vi "X.vi"(9 "X(k-1)":dbl=0.1, 10 "Ýterasyon Denge":dbl, 11 "denge degeri":dbl) -> (0 "error":bool, 2 "output X(k-1)":dbl=0.1, 3 "output x 1":dbl, 4 "cycle":bool)   [LabVIEW 2014]
uses:
  Sub_VI/show_sensitivity.vi
  Sub_VI/global get findinput.vi
  DB_Global_4_kart-Test.vi
panel:
  out "cycle 2":bool
  in  "GPIB In":refnum<visa-resource-name>="GPIB0::8::INSTR"
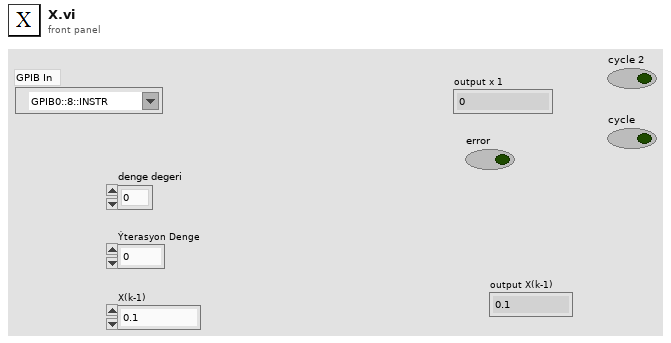
[diagram p1: front panel]
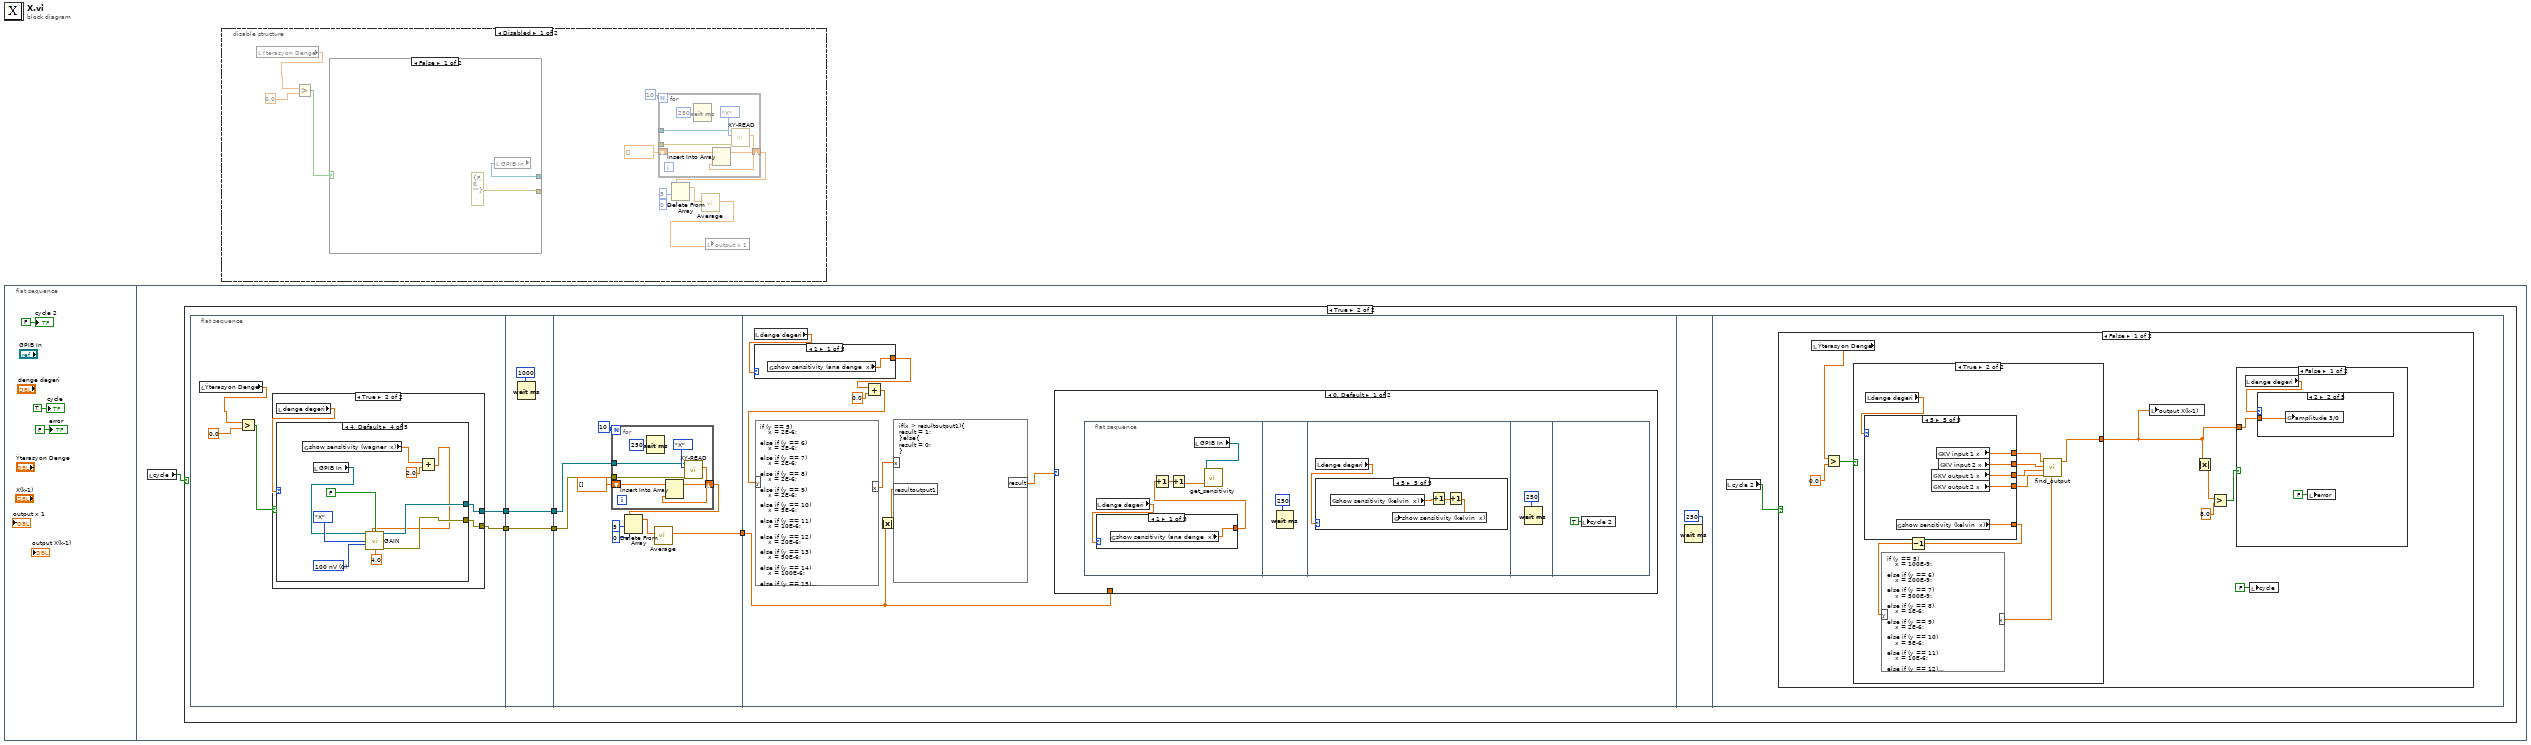
[diagram p0: block diagram]
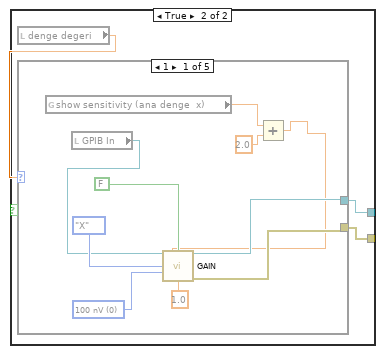
[diagram p2: hidden frame]
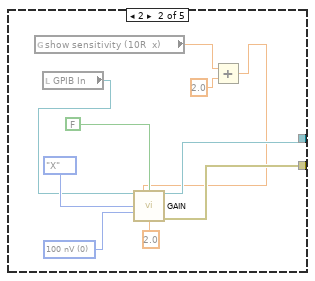
[diagram p3: hidden frame]
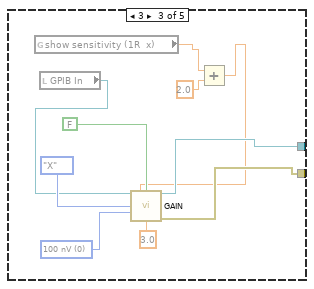
[diagram p4: hidden frame]
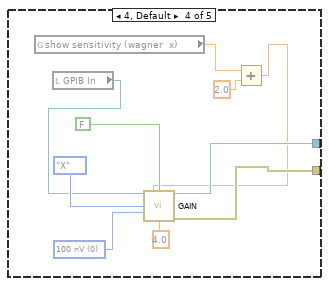
[diagram p5: hidden frame]
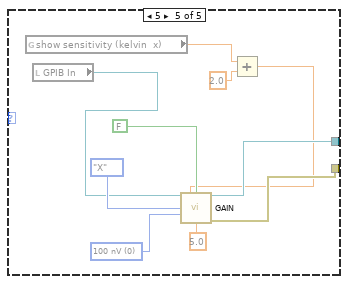
[diagram p6: hidden frame]
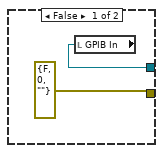
[diagram p9: hidden frame]
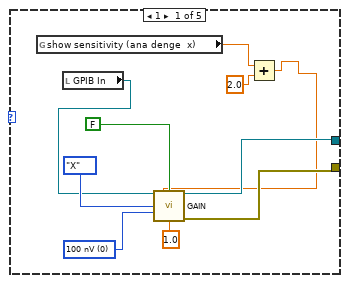
[diagram p10: hidden frame]
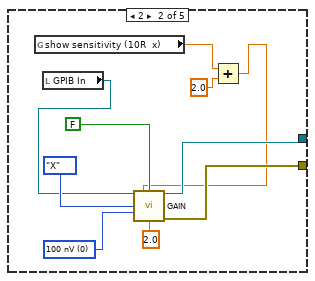
[diagram p11: hidden frame]
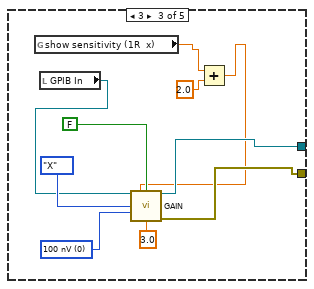
[diagram p12: hidden frame]
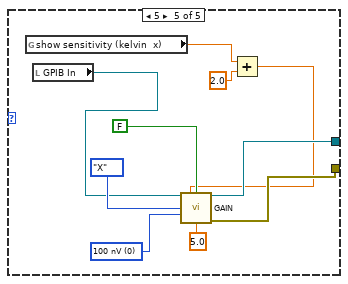
[diagram p13: hidden frame]
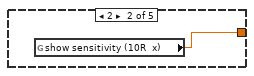
[diagram p14: hidden frame]
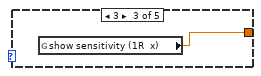
[diagram p15: hidden frame]
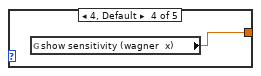
[diagram p16: hidden frame]
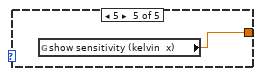
[diagram p17: hidden frame]
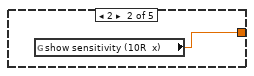
[diagram p18: hidden frame]
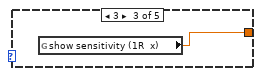
[diagram p19: hidden frame]
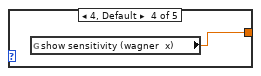
[diagram p20: hidden frame]
diagram:
  n1 = flat-sequence {
    frame #0 {
      "error" <- FALSE ("error")
      "cycle" <- TRUE ("error")
      "cycle 2" <- FALSE ("error")
    }
    frame #1 {
      n2 = local read "cycle"() -> (w4:bool)
      n3 = case shown="True" w4 {
        frame False {
        }
        frame True {
          n4 = flat-sequence {
            tunnel: [w11] -> w8
            tunnel: [w10] -> w6
            tunnel: [w71] -> w9
            tunnel: w8 -> [w71]
            tunnel: [w70] -> w7
            tunnel: w6 -> [w70]
            tunnel: w9 -> [w75]
            tunnel: w7 -> [w74]
            tunnel: [w73] -> w5
            tunnel: w5 -> [w92]
            frame #0 {
              n5 = local read "Ýterasyon Denge"() -> (w12:dbl)
              n6 = Greater?(x=w12, y=0.0) -> (0:w13:bool)
              n7 = case shown="True" w13 {
                tunnel: [w16 w18] -> w11
                tunnel: [errorcluster {"status"=FALSE, "code"=0, "source"=""} ("error out") w17] -> w10
                frame False {
                  n8 = local read "GPIB In"() -> (w16:refnum<visa-resource-name>)
                }
                frame True {
                  n9 = local read "denge degeri"() -> (w19:dbl)
                  n10 = case shown="4, Default" w19 {
                    tunnel: [w24 w34 w44 w54 w65] -> w18
                    tunnel: [w23 w33 w43 w53 w64] -> w17
                    frame 1 {
                      w26 = u16 0 items=["100 nV", "200 nV", "500 nV", "1 uV", "2 uV", "5 uV", "10 uV", "20 uV", "50 uV", "100 uV", "200 uV", "500 uV", "1 mV"] ("Min. Hassasiyet")
                      n11 = global read "show_sensitivity.vi" "show sensitivity (ana denge  x)"() -> (w21:dbl)
                      n12 = local read "GPIB In"() -> (w27:refnum<visa-resource-name>)
                      n13 = Add(x=w21, y=2.0) -> (x+y=w20:dbl)
                      n14 = call "GAIN.vi"("SR850 GPIB In"=w27, "Max. Hassasiyet"=w20, "Auto Gain (False)"=FALSE, "Enum"=enum16{"X", "Y"}."X", "Min. Hassasiyet"=w26, "choose"=1.0) -> ("SR850 GPIB Out"=w24:refnum<visa-resource-name>, "error out"=w23:errorcluster)  [unwired: 7 in, 1 out]
                    }
                    frame 2 {
                      w36 = u16 0 items=["100 nV", "200 nV", "500 nV", "1 uV", "2 uV", "5 uV", "10 uV", "20 uV", "50 uV", "100 uV", "200 uV", "500 uV", "1 mV"] ("Min. Hassasiyet")
                      n15 = global read "show_sensitivity.vi" "show sensitivity (10R  x)"() -> (w30:dbl)
                      n16 = local read "GPIB In"() -> (w37:refnum<visa-resource-name>)
                      n17 = Add(x=w30, y=2.0) -> (x+y=w31:dbl)
                      n18 = call "GAIN.vi"("SR850 GPIB In"=w37, "Max. Hassasiyet"=w31, "Auto Gain (False)"=FALSE, "Enum"=enum16{"X", "Y"}."X", "Min. Hassasiyet"=w36, "choose"=2.0) -> ("SR850 GPIB Out"=w34:refnum<visa-resource-name>, "error out"=w33:errorcluster)  [unwired: 7 in, 1 out]
                    }
                    frame 3 {
                      w46 = u16 0 items=["100 nV", "200 nV", "500 nV", "1 uV", "2 uV", "5 uV", "10 uV", "20 uV", "50 uV", "100 uV", "200 uV", "500 uV", "1 mV"] ("Min. Hassasiyet")
                      n19 = global read "show_sensitivity.vi" "show sensitivity (1R  x)"() -> (w41:dbl)
                      n20 = local read "GPIB In"() -> (w47:refnum<visa-resource-name>)
                      n21 = Add(x=w41, y=2.0) -> (x+y=w40:dbl)
                      n22 = call "GAIN.vi"("SR850 GPIB In"=w47, "Max. Hassasiyet"=w40, "Auto Gain (False)"=FALSE, "Enum"=enum16{"X", "Y"}."X", "Min. Hassasiyet"=w46, "choose"=3.0) -> ("SR850 GPIB Out"=w44:refnum<visa-resource-name>, "error out"=w43:errorcluster)  [unwired: 7 in, 1 out]
                    }
                    frame 4, Default {
                      w56 = u16 0 items=["100 nV", "200 nV", "500 nV", "1 uV", "2 uV", "5 uV", "10 uV", "20 uV", "50 uV", "100 uV", "200 uV", "500 uV", "1 mV"] ("Min. Hassasiyet")
                      n23 = global read "show_sensitivity.vi" "show sensitivity (wagner  x)"() -> (w51:dbl)
                      n24 = local read "GPIB In"() -> (w57:refnum<visa-resource-name>)
                      n25 = Add(x=w51, y=2.0) -> (x+y=w50:dbl)
                      n26 = call "GAIN.vi"("SR850 GPIB In"=w57, "Max. Hassasiyet"=w50, "Auto Gain (False)"=FALSE, "Enum"=enum16{"X", "Y"}."X", "Min. Hassasiyet"=w56, "choose"=4.0) -> ("SR850 GPIB Out"=w54:refnum<visa-resource-name>, "error out"=w53:errorcluster)  [unwired: 7 in, 1 out]
                    }
                    frame 5 {
                      w67 = u16 0 items=["100 nV", "200 nV", "500 nV", "1 uV", "2 uV", "5 uV", "10 uV", "20 uV", "50 uV", "100 uV", "200 uV", "500 uV", "1 mV"] ("Min. Hassasiyet")
                      n27 = global read "show_sensitivity.vi" "show sensitivity (kelvin  x)"() -> (w60:dbl)
                      n28 = local read "GPIB In"() -> (w63:refnum<visa-resource-name>)
                      n29 = Add(x=w60, y=2.0) -> (x+y=w61:dbl)
                      n30 = call "GAIN.vi"("SR850 GPIB In"=w63, "Max. Hassasiyet"=w61, "Auto Gain (False)"=FALSE, "Enum"=enum16{"X", "Y"}."X", "Min. Hassasiyet"=w67, "choose"=5.0) -> ("SR850 GPIB Out"=w65:refnum<visa-resource-name>, "error out"=w64:errorcluster)  [unwired: 7 in, 1 out]
                    }
                  }
                }
              }
            }
            frame #1 {
              n31 = Wait (ms)(milliseconds to wait=u32 1000) -> ()  [unwired: 1 out]
            }
            frame #2 {
              n32 = for {
                N: 10 -> [_]
                tunnel: w75 -> [w87]
                tunnel: w74 -> [w86]
                shift-right: [w83] -> w79
                shift-left: dbl[] [] -> [w84]
                n33 = Wait (ms)(milliseconds to wait=u32 250) -> ()  [unwired: 1 out]
                n34 = call "XY-READ.vi"("Error IN"=w86, "X/Y ?"=enum16{"X", "Y"}."X" ("Enum"), "SR850 GPIB IN"=w87) -> ("SR850_Reading"=w85:dbl)  [unwired: 6 in, 2 out]
                n35 = Insert Into Array(array=w84, new element=w85) -> (w83:dbl[])  [unwired: 1 in]
              }
              n36 = Delete From Array(array=w79, length=5, index=0) -> (array with subset deleted=w78:dbl[])  [unwired: 1 out]
              n37 = call "Average.vi"("Array"=w78) -> ("Average"=w73:dbl)  [unwired: 9 in, 1 out]
            }
            frame #3 {
              n38 = local read "denge degeri"() -> (w91:dbl)
              n39 = case shown="1" w91 {
                tunnel: [w97 w98 w99 w100 w101] -> w90
                frame 1 {
                  n40 = global read "show_sensitivity.vi" "show sensitivity (ana denge  x)"() -> (w97:dbl)
                }
                frame 2 {
                  n41 = global read "show_sensitivity.vi" "show sensitivity (10R  x)"() -> (w98:dbl)
                }
                frame 3 {
                  n42 = global read "show_sensitivity.vi" "show sensitivity (1R  x)"() -> (w99:dbl)
                }
                frame 4, Default {
                  n43 = global read "show_sensitivity.vi" "show sensitivity (wagner  x)"() -> (w100:dbl)
                }
                frame 5 {
                  n44 = global read "show_sensitivity.vi" "show sensitivity (kelvin  x)"() -> (w101:dbl)
                }
              }
              n45 = Add(x=w90, y=0.0) -> (x+y=w94:dbl)
              n46 = formula code="if (y == 5) \n    x = 2E-6;\n\nelse if (y == 6) \n    x = 2E-6;\n\nelse if (y == 7) \n    x = 2E-6;\n\nelse if (y == 8) \n    x = 2E-6;\n\nelse if (y == 9) \n    x = 2E-6;\n\nelse if (y == 10) \n    x = 5E-6;\n\nelse if (y == 11) \n    x = 10E-6;\n\nelse if (y == 12) \n    x = 20E-6;\n\nelse if (y == 13) \n    x = 50E-6;\n\nelse if (y == 14) \n    x = 100E-6;\n\nelse if (y == 15) \n    x = 200E-6;\n\nelse if (y == 16) \n    x = 500E-6;\n\nelse if (y == 17) \n    x = 1E-3;\n\nelse if (y == 18) \n    x = 2E-3;\n\nelse if (y == 19) \n    x = 5E-3;\n\nelse if (y == 20) \n    x = 10E-3;\n\nelse if (y == 21) \n    x = 20E-3;\n\nelse if (y == 22) \n    x = 50E-3;\n\nelse if (y == 23) \n    x = 100E-3;\n\nelse if (y == 24) \n    x = 200E-3;\n\nelse if (y == 25) \n    x = 500E-3;\n\nelse if (y == 26) \n    x = 1;\n\nelse \n    x = 1;"("y"=w94) -> ("x"=w96:dbl)
              n47 = Absolute Value(x=w92) -> (abs(x)=w89:dbl)
              n48 = formula code="if(x > resultoutput1){\nresult = 1;\n}else{\nresult = 0;\n}"("x"=w96, "resultoutput1"=w89) -> ("result"=w93:dbl)
              n49 = case shown="0, Default" w93 {
                tunnel: w92 -> [_ w131]
                frame 0, Default {
                  n50 = flat-sequence {
                    frame #0 {
                      n51 = local read "denge degeri"() -> (w104:dbl)
                      n52 = case shown="1" w104 {
                        tunnel: [w107 w108 w109 w110 w111] -> w103
                        frame 1 {
                          n53 = global read "show_sensitivity.vi" "show sensitivity (ana denge  x)"() -> (w107:dbl)
                        }
                        frame 2 {
                          n54 = global read "show_sensitivity.vi" "show sensitivity (10R  x)"() -> (w108:dbl)
                        }
                        frame 3 {
                          n55 = global read "show_sensitivity.vi" "show sensitivity (1R  x)"() -> (w109:dbl)
                        }
                        frame 4, Default {
                          n56 = global read "show_sensitivity.vi" "show sensitivity (wagner  x)"() -> (w110:dbl)
                        }
                        frame 5 {
                          n57 = global read "show_sensitivity.vi" "show sensitivity (kelvin  x)"() -> (w111:dbl)
                        }
                      }
                      n58 = Increment(x=w103) -> (x+1=w102:dbl)
                      n59 = Increment(x=w102) -> (x+1=w105:dbl)
                      n60 = local read "GPIB In"() -> (w106:refnum<visa-resource-name>)
                      n61 = call "get_sensitivity.vi"("input 1"=w105, "SR850 GPIB In"=w106) -> ()  [unwired: 8 in, 2 out]
                    }
                    frame #1 {
                      n62 = Wait (ms)(milliseconds to wait=u32 250) -> ()  [unwired: 1 out]
                    }
                    frame #2 {
                      n63 = local read "denge degeri"() -> (w113:dbl)
                      n64 = case shown="5" w113 {
                        frame 1 {
                          n65 = global read "show_sensitivity.vi" "show sensitivity (ana denge  x)"() -> (w116:dbl)
                          n66 = Increment(x=w116) -> (x+1=w115:dbl)
                          n67 = Increment(x=w115) -> (x+1=w114:dbl)
                          n68 = global write "show_sensitivity.vi" "show sensitivity (ana denge  x)"(w114) -> ()
                        }
                        frame 2 {
                          n69 = global read "show_sensitivity.vi" "show sensitivity (10R  x)"() -> (w119:dbl)
                          n70 = Increment(x=w119) -> (x+1=w118:dbl)
                          n71 = Increment(x=w118) -> (x+1=w117:dbl)
                          n72 = global write "show_sensitivity.vi" "show sensitivity (10R  x)"(w117) -> ()
                        }
                        frame 3 {
                          n73 = global read "show_sensitivity.vi" "show sensitivity (1R  x)"() -> (w122:dbl)
                          n74 = Increment(x=w122) -> (x+1=w121:dbl)
                          n75 = Increment(x=w121) -> (x+1=w120:dbl)
                          n76 = global write "show_sensitivity.vi" "show sensitivity (1R  x)"(w120) -> ()
                        }
                        frame 4, Default {
                          n77 = global read "show_sensitivity.vi" "show sensitivity (wagner  x)"() -> (w125:dbl)
                          n78 = Increment(x=w125) -> (x+1=w124:dbl)
                          n79 = Increment(x=w124) -> (x+1=w123:dbl)
                          n80 = global write "show_sensitivity.vi" "show sensitivity (wagner  x)"(w123) -> ()
                        }
                        frame 5 {
                          n81 = global read "show_sensitivity.vi" "show sensitivity (kelvin  x)"() -> (w128:dbl)
                          n82 = Increment(x=w128) -> (x+1=w127:dbl)
                          n83 = Increment(x=w127) -> (x+1=w126:dbl)
                          n84 = global write "show_sensitivity.vi" "show sensitivity (kelvin  x)"(w126) -> ()
                        }
                      }
                    }
                    frame #3 {
                      n85 = Wait (ms)(milliseconds to wait=u32 250) -> ()  [unwired: 1 out]
                    }
                    frame #4 {
                      n86 = local write "cycle 2"(TRUE ("cycle")) -> ()
                    }
                  }
                }
                frame 1 {
                  n87 = local write "output x 1"(w131) -> ()
                  n88 = local write "cycle 2"(FALSE ("cycle")) -> ()
                }
              }
            }
            frame #4 {
              n89 = Wait (ms)(milliseconds to wait=u32 250) -> ()  [unwired: 1 out]
            }
            frame #5 {
              n90 = local read "cycle 2"() -> (w134:bool)
              n91 = case shown="False" w134 {
                frame False {
                  n92 = local read "Ýterasyon Denge"() -> (w136:dbl)
                  n93 = Greater?(x=w136, y=0.0) -> (0:w138:bool)
                  n94 = case shown="True" w138 {
                    tunnel: [w143 w151] -> w139
                    frame False {
                      n95 = local read "X(k-1)"() -> (w143:dbl)
                    }
                    frame True {
                      n96 = local read "denge degeri"() -> (w152:dbl)
                      n97 = case shown="5" w152 {
                        tunnel: [w157 w162 w167 w172 w177] -> w150
                        tunnel: [w156 w161 w166 w171 w176] -> w149
                        tunnel: [w155 w160 w165 w170 w175] -> w148
                        tunnel: [w154 w159 w164 w169 w174] -> w147
                        tunnel: [w153 w158 w163 w168 w173] -> w146
                        frame 1 {
                          n98 = global read "show_sensitivity.vi" "show sensitivity (ana denge  x)"() -> (w153:dbl)
                          n99 = global read "global get findinput.vi" "AD output 1 x"() -> (w155:dbl)
                          n100 = global read "global get findinput.vi" "AD output 2 x"() -> (w154:dbl)
                          n101 = global read "global get findinput.vi" "AD input 1 x"() -> (w157:dbl)
                          n102 = global read "global get findinput.vi" "AD input 2 x"() -> (w156:dbl)
                        }
                        frame 2 {
                          n103 = global read "show_sensitivity.vi" "show sensitivity (10R  x)"() -> (w158:dbl)
                          n104 = global read "global get findinput.vi" "10R output 1 x"() -> (w160:dbl)
                          n105 = global read "global get findinput.vi" "10R output 2 x"() -> (w159:dbl)
                          n106 = global read "global get findinput.vi" "10R input 2 x"() -> (w161:dbl)
                          n107 = global read "global get findinput.vi" "10R input 1 x"() -> (w162:dbl)
                        }
                        frame 3 {
                          n108 = global read "show_sensitivity.vi" "show sensitivity (1R  x)"() -> (w163:dbl)
                          n109 = global read "global get findinput.vi" "1R output 2 x"() -> (w164:dbl)
                          n110 = global read "global get findinput.vi" "1R output 1 x"() -> (w165:dbl)
                          n111 = global read "global get findinput.vi" "1R input 2 x"() -> (w166:dbl)
                          n112 = global read "global get findinput.vi" "1R input 1 x"() -> (w167:dbl)
                        }
                        frame 4, Default {
                          n113 = global read "show_sensitivity.vi" "show sensitivity (wagner  x)"() -> (w168:dbl)
                          n114 = global read "global get findinput.vi" "W output 1 x"() -> (w170:dbl)
                          n115 = global read "global get findinput.vi" "W output 2 x"() -> (w169:dbl)
                          n116 = global read "global get findinput.vi" "W input 1 x"() -> (w172:dbl)
                          n117 = global read "global get findinput.vi" "W input 2 x"() -> (w171:dbl)
                        }
                        frame 5 {
                          n118 = global read "show_sensitivity.vi" "show sensitivity (kelvin  x)"() -> (w173:dbl)
                          n119 = global read "global get findinput.vi" "KV output 1 x"() -> (w175:dbl)
                          n120 = global read "global get findinput.vi" "KV output 2 x"() -> (w174:dbl)
                          n121 = global read "global get findinput.vi" "KV input 1 x"() -> (w177:dbl)
                          n122 = global read "global get findinput.vi" "KV input 2 x"() -> (w176:dbl)
                        }
                      }
                      n123 = Decrement(x=w146) -> (x-1=w144:dbl)
                      n124 = formula code="if (y == 5) \n    x = 100E-9;\n\nelse if (y == 6) \n    x = 200E-9;\n\nelse if (y == 7) \n    x = 500E-9;\n\nelse if (y == 8) \n    x = 1E-6;\n\nelse if (y == 9) \n    x = 2E-6;\n\nelse if (y == 10) \n    x = 5E-6;\n\nelse if (y == 11) \n    x = 10E-6;\n\nelse if (y == 12) \n    x = 20E-6;\n\nelse if (y == 13) \n    x = 50E-6;\n\nelse if (y == 14) \n    x = 100E-6;\n\nelse if (y == 15) \n    x = 200E-6;\n\nelse if (y == 16) \n    x = 500E-6;\n\nelse if (y == 17) \n    x = 1E-3;\n\nelse if (y == 18) \n    x = 2E-3;\n\nelse if (y == 19) \n    x = 5E-3;\n\nelse if (y == 20) \n    x = 10E-3;\n\nelse if (y == 21) \n    x = 20E-3;\n\nelse if (y == 22) \n    x = 50E-3;\n\nelse if (y == 23) \n    x = 100E-3;\n\nelse if (y == 24) \n    x = 200E-3;\n\nelse if (y == 25) \n    x = 500E-3;\n\nelse if (y == 26) \n    x = 1;\n\nelse \n    x = 1;"("y"=w144) -> ("x"=w145:dbl)
                      n125 = call "find_output.vi"("find output"=w145, "output 2"=w147, "output 1"=w148, "input 2"=w149, "input 1"=w150) -> ("getInput"=w151:dbl)  [unwired: 6 in]
                    }
                  }
                  n126 = local write "output X(k-1)"(w139) -> ()
                  n127 = Absolute Value(x=w139) -> (abs(x)=w140:dbl)
                  n128 = Greater?(x=w140, y=8.0 ("Wagner  X(k-1)")) -> (0:w142:bool)
                  n129 = case shown="False" w142 {
                    tunnel: w139 -> [w179 _]
                    frame False {
                      n130 = local read "denge degeri"() -> (w180:dbl)
                      n131 = case shown="2" w180 {
                        tunnel: w179 -> [w181 w182 w183 w184 w185]
                        frame 1 {
                          n132 = global write "DB_Global_4_kart-Test.vi" "amplitude 2/0"(w181) -> ()
                        }
                        frame 2 {
                          n133 = global write "DB_Global_4_kart-Test.vi" "amplitude 3/0"(w182) -> ()
                        }
                        frame 3 {
                          n134 = global write "DB_Global_4_kart-Test.vi" "amplitude 3/1"(w183) -> ()
                        }
                        frame 4, Default {
                          n135 = global write "DB_Global_4_kart-Test.vi" "amplitude 1/1"(w184) -> ()
                        }
                        frame 5 {
                          n136 = global write "DB_Global_4_kart-Test.vi" "amplitude 2/1"(w185) -> ()
                        }
                      }
                      n137 = local write "error"(FALSE ("error")) -> ()
                    }
                    frame True {
                      n138 = local write "error"(TRUE ("error")) -> ()
                    }
                  }
                  n139 = local write "cycle"(FALSE ("cycle")) -> ()
                }
                frame True {
                  n140 = local write "cycle"(TRUE ("cycle")) -> ()
                }
              }
            }
          }
        }
      }
    }
  }
  n141 = disable-structure shown="Disabled" {
    frame Disabled {
      n142 = local read "Ýterasyon Denge"() -> (w190:dbl)
      n143 = Greater?(x=w190, y=0.0) -> (0:w189:bool)
      n144 = case shown="False" w189 {
        tunnel: [w201 w203] -> _
        tunnel: [errorcluster {"status"=FALSE, "code"=0, "source"=""} ("error out") w202] -> _
        frame False {
          n145 = local read "GPIB In"() -> (w201:refnum<visa-resource-name>)
        }
        frame True {
          n146 = local read "denge degeri"() -> (w204:dbl)
          n147 = case shown="1" w204 {
            tunnel: [w209 w219 w229 w239 w250] -> w203
            tunnel: [w208 w218 w228 w238 w249] -> w202
            frame 1 {
              w211 = u16 0 items=["100 nV", "200 nV", "500 nV", "1 uV", "2 uV", "5 uV", "10 uV", "20 uV", "50 uV", "100 uV", "200 uV", "500 uV", "1 mV"] ("Min. Hassasiyet")
              n148 = global read "show_sensitivity.vi" "show sensitivity (ana denge  x)"() -> (w206:dbl)
              n149 = local read "GPIB In"() -> (w212:refnum<visa-resource-name>)
              n150 = Add(x=w206, y=2.0) -> (x+y=w205:dbl)
              n151 = call "GAIN.vi"("SR850 GPIB In"=w212, "Max. Hassasiyet"=w205, "Auto Gain (False)"=FALSE, "Enum"=enum16{"X", "Y"}."X", "Min. Hassasiyet"=w211, "choose"=1.0) -> ("SR850 GPIB Out"=w209:refnum<visa-resource-name>, "error out"=w208:errorcluster)  [unwired: 7 in, 1 out]
            }
            frame 2 {
              w221 = u16 0 items=["100 nV", "200 nV", "500 nV", "1 uV", "2 uV", "5 uV", "10 uV", "20 uV", "50 uV", "100 uV", "200 uV", "500 uV", "1 mV"] ("Min. Hassasiyet")
              n152 = global read "show_sensitivity.vi" "show sensitivity (10R  x)"() -> (w215:dbl)
              n153 = local read "GPIB In"() -> (w222:refnum<visa-resource-name>)
              n154 = Add(x=w215, y=2.0) -> (x+y=w216:dbl)
              n155 = call "GAIN.vi"("SR850 GPIB In"=w222, "Max. Hassasiyet"=w216, "Auto Gain (False)"=FALSE, "Enum"=enum16{"X", "Y"}."X", "Min. Hassasiyet"=w221, "choose"=2.0) -> ("SR850 GPIB Out"=w219:refnum<visa-resource-name>, "error out"=w218:errorcluster)  [unwired: 7 in, 1 out]
            }
            frame 3 {
              w231 = u16 0 items=["100 nV", "200 nV", "500 nV", "1 uV", "2 uV", "5 uV", "10 uV", "20 uV", "50 uV", "100 uV", "200 uV", "500 uV", "1 mV"] ("Min. Hassasiyet")
              n156 = global read "show_sensitivity.vi" "show sensitivity (1R  x)"() -> (w226:dbl)
              n157 = local read "GPIB In"() -> (w232:refnum<visa-resource-name>)
              n158 = Add(x=w226, y=2.0) -> (x+y=w225:dbl)
              n159 = call "GAIN.vi"("SR850 GPIB In"=w232, "Max. Hassasiyet"=w225, "Auto Gain (False)"=FALSE, "Enum"=enum16{"X", "Y"}."X", "Min. Hassasiyet"=w231, "choose"=3.0) -> ("SR850 GPIB Out"=w229:refnum<visa-resource-name>, "error out"=w228:errorcluster)  [unwired: 7 in, 1 out]
            }
            frame 4, Default {
              w241 = u16 0 items=["100 nV", "200 nV", "500 nV", "1 uV", "2 uV", "5 uV", "10 uV", "20 uV", "50 uV", "100 uV", "200 uV", "500 uV", "1 mV"] ("Min. Hassasiyet")
              n160 = global read "show_sensitivity.vi" "show sensitivity (wagner  x)"() -> (w236:dbl)
              n161 = local read "GPIB In"() -> (w242:refnum<visa-resource-name>)
              n162 = Add(x=w236, y=2.0) -> (x+y=w235:dbl)
              n163 = call "GAIN.vi"("SR850 GPIB In"=w242, "Max. Hassasiyet"=w235, "Auto Gain (False)"=FALSE, "Enum"=enum16{"X", "Y"}."X", "Min. Hassasiyet"=w241, "choose"=4.0) -> ("SR850 GPIB Out"=w239:refnum<visa-resource-name>, "error out"=w238:errorcluster)  [unwired: 7 in, 1 out]
            }
            frame 5 {
              w252 = u16 0 items=["100 nV", "200 nV", "500 nV", "1 uV", "2 uV", "5 uV", "10 uV", "20 uV", "50 uV", "100 uV", "200 uV", "500 uV", "1 mV"] ("Min. Hassasiyet")
              n164 = global read "show_sensitivity.vi" "show sensitivity (kelvin  x)"() -> (w245:dbl)
              n165 = local read "GPIB In"() -> (w248:refnum<visa-resource-name>)
              n166 = Add(x=w245, y=2.0) -> (x+y=w246:dbl)
              n167 = call "GAIN.vi"("SR850 GPIB In"=w248, "Max. Hassasiyet"=w246, "Auto Gain (False)"=FALSE, "Enum"=enum16{"X", "Y"}."X", "Min. Hassasiyet"=w252, "choose"=5.0) -> ("SR850 GPIB Out"=w250:refnum<visa-resource-name>, "error out"=w249:errorcluster)  [unwired: 7 in, 1 out]
            }
          }
        }
      }
      n168 = for {
        N: 10 -> [_]
        tunnel: [w260] -> w192
        tunnel: [w259] -> w191
        shift-right: [w256] -> w195
        shift-left: dbl[] [] -> [w257]
        n169 = Wait (ms)(milliseconds to wait=u32 250) -> ()  [unwired: 1 out]
        n170 = call "XY-READ.vi"("Error IN"=w259, "X/Y ?"=enum16{"X", "Y"}."X" ("Enum"), "SR850 GPIB IN"=w260) -> ("SR850_Reading"=w258:dbl)  [unwired: 6 in, 2 out]
        n171 = Insert Into Array(array=w257, new element=w258) -> (w256:dbl[])  [unwired: 1 in]
      }
      n172 = Delete From Array(array=w195, length=5, index=0) -> (array with subset deleted=w196:dbl[])  [unwired: 1 out]
      n173 = call "Average.vi"("Array"=w196) -> ("Average"=w199:dbl)  [unwired: 9 in, 1 out]
      n174 = local write "output x 1"(w199) -> ()
    }
    frame Enabled {
    }
  }
